vi "PPG_ABC.destructor.vi"(0 "i ref in":refnum<vi>, 5 "error in(no error)":errorcluster) -> (19 "error out":errorcluster)   [LabVIEW 2014, in "PPG_ABC.lvlib"]
doc: "This is the destructor of a class.\n\nLicense Agreement for this software:\n\nCopyright (C)\nGesellschaft für Schwerionenforschung, GSI\nPlanckstr. 1\n64291 Darmstadt\nGermany\n\nContact: D.Beck@gsi.de \n\nThis program is free software; you can redistribute it and/or modify it under the terms of the \nGNU General Public License as published by the Free Software Foundation; either version 2 of \nthe license, or (at your option) any later version.\n\nThis program is distributed in the hope that it will be useful, but WITHOUT ANY WARRANTY; \nwithout even the implied warranty of MERCHANTABILITY or FITNESS FOR A PARTICULAR PURPOSE. See the GNU General License for more details (http://www.gnu.org).\n\nGesellschaft für Schwerionenforschung, GSI\nPlanckstr. 1, 64291 Darmstadt, Germany\nFor all questions and ideas contact: M.Richter@gsi.de, H.Brand@gsi.de or D.Beck@gsi.de.\nLast update: 16-JUN-2004"
uses:
  PPG_ABC.lvlib
  NI_FPGA_PPG/NI_FPGA_PPG.lvlib
  CSlibraries-extern/DimLVEvent/LVDimInterface/LVDimInterface.lvlib
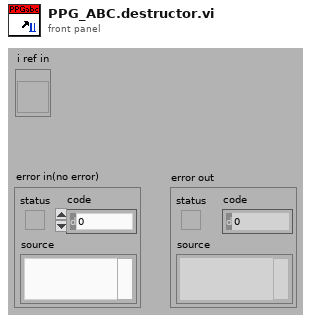
[diagram p1: front panel]
types:
  T1 = typedef "PPG_ABC.lvlib/PPG_ABC.i attribute.ctl" = cluster{"patternGroups":T2[], "defaultLetter":string, "defaultPatternGroup":i32, "PGRunning":T3, "PGRunningID":i32, "pgStarting":T4}
  T2 = typedef "PPG_ABC.lvlib/PPG_ABC.PG_dataType.ctl" = cluster{"PGDevice":string, "rawPatternData":cluster{"triggerCondition":i32, "timeTable":dbl[], "channelTable":string[]}[]}
  T3 = typedef "PPG_ABC.lvlib/PPG_ABC.PG_Running.ctl" = i32
  T4 = typedef "Semaphore RefNum" = refnum<k1>
  T5 = enum16{"SetAttribute", "GetAttribute", "CreateAttribute", "DestroyAttribute", "DestroyAllAtributes"}
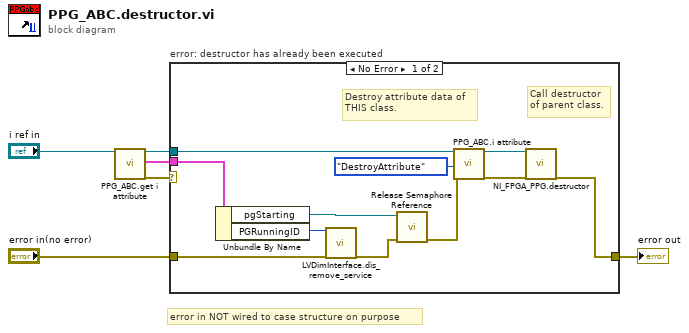
[diagram p0: block diagram]
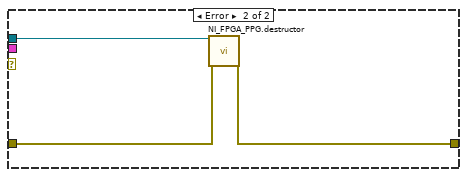
[diagram p2: hidden frame]
diagram:
  # "error in NOT wired to case structure on purpose"
  n1 = call "PPG_ABC.get i attribute.vi"("i ref in"="i ref in") -> ("i ref out"=w2:refnum<vi>, "i attribute"=w1:T1, "error out"=w3:errorcluster)  [unwired: 16 in]
  n2 = case "error: destructor has already been executed" shown="No Error" w3 {
    tunnel: [w14 w18] -> w6
    tunnel: "error in(no error)" -> [w10 w19]
    tunnel: w2 -> [w13 w20]
    tunnel: w1 -> [w12 _]
    frame No Error {
      # "Destroy attribute data of \nTHIS class."
      # "Call destructor\nof parent class."
      n3 = Unbundle By Name(w12) -> ("pgStarting"=w9:T4, "PGRunningID"=w11:i32)
      n4 = call "LVDimInterface.dis_remove_service.vi"("my_serviceID"=w11, "error in (no error)"=w10) -> ("error out"=w8:errorcluster)  [unwired: 17 in]
      n5 = call <vilib>:"Release Semaphore Reference.vi"("error in (no error)"=w8, "semaphore"=w9) -> ("error out"=w7:errorcluster)  [unwired: 8 in, 1 out]
      n6 = call "PPG_ABC.i attribute.vi"("VI Refnum"=w13, "Action"=T5."DestroyAttribute", "error in (no error)"=w7) -> ("VI Refnum out"=w16:refnum<vi>, "error out"=w15:errorcluster)  [unwired: 14 in, 1 out]
      n7 = call "NI_FPGA_PPG.destructor.vi"("i ref in"=w16, "error in (no error)"=w15) -> ("error out"=w14:errorcluster)  [unwired: 17 in]
    }
    frame Error {
      n8 = call "NI_FPGA_PPG.destructor.vi"("i ref in"=w20, "error in (no error)"=w19) -> ("error out"=w18:errorcluster)  [unwired: 17 in]
    }
  }
  "error out" <- w6
